vi "Read Analog Output Configuration.vi"(8 "error in (no error)":errorcluster, 11 "VGC in":refnum<class "PL Inficon VGC.lvclass">) -> (0 "error out":errorcluster, 1 "characteristic":u16(ring) items=["log", "log a", "log -6", "log -3", "log +0", "log +3", "log c1", "log c2", "log c3", "lin -10", "lin -9", "lin -8", "lin -7", "lin -6", "lin -5", "lin -4", "lin -3", "lin -2", "lin -1", "lin +0", "lin +1", "lin +2", "lin +3", "IM221", "log c4", "PM411", "ch x", "PRM10K", "IMR110", "IMR120", "IMR310", "IMR320"], 2 "channel":u16(ring) items=["channel 1", "channel 2", "channel 3"], 3 "VGC out":refnum<class "PL Inficon VGC.lvclass">)   [LabVIEW 2015, in "PL Inficon VGC.lvclass"]
doc: "Reads analog output configuration ."
uses:
  PL Inficon VGC.lvclass
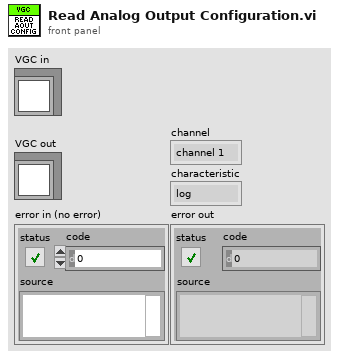
[diagram p1: front panel]
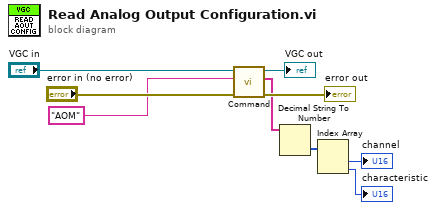
[diagram p0: block diagram]
diagram:
  n1 = call "Command.vi"("error in (no error)"="error in (no error)", "command"="AOM" ("format string"), "VGC in"="VGC in") -> ("error out"=→"error out":errorcluster, "response data"=w4:string[], "VGC out"=→"VGC out":refnum<class "PL Inficon VGC.lvclass">)  [unwired: 6 in]
  n2 = Decimal String To Number(string=w4) -> (number=w5:i32[])  [unwired: 2 in, 1 out]
  n3 = Index Array(array=w5) -> (element #1=→"channel":i32, element #2=→"characteristic":i32)  [unwired: 2 in]
